vi "Act On Test.vi"(6 "Report Action":T1, 8 "error in":errorcluster, 9 "Values":variant[](array[variant]), 10 "Parameters":string[](array[string]), 11 "TDMS in":refnum<class "TDMS.lvclass">) -> (0 "error out":errorcluster, 3 "TDMS out":refnum<class "TDMS.lvclass">)   [LabVIEW 2019, in "TDMS.lvlib" / "TDMS.lvclass"]
uses:
  TDMS.lvclass
  builds/Tools/Report.lvlibp/Custom Controls/Report Action.ctl
  TDMS.lvclass/TDMS.ctl
  builds/Tools/Report.lvlibp/Report.lvclass
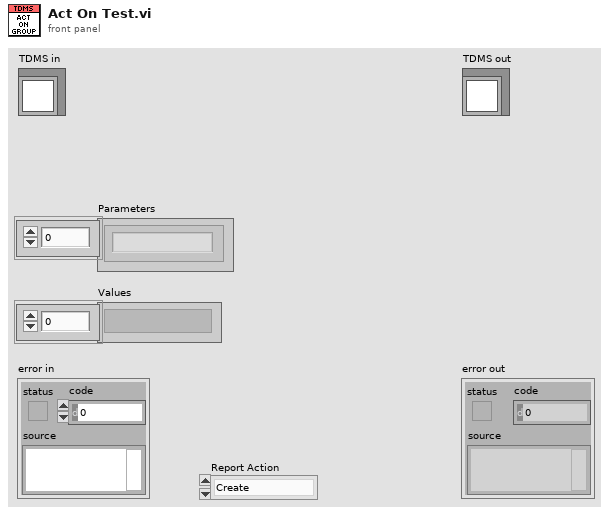
[diagram p1: front panel]
types:
  T1 = typedef "Report.lvlibp/Report.lvclass/Report Action.ctl" = enum16{"Create", "Append", "Destroy"}
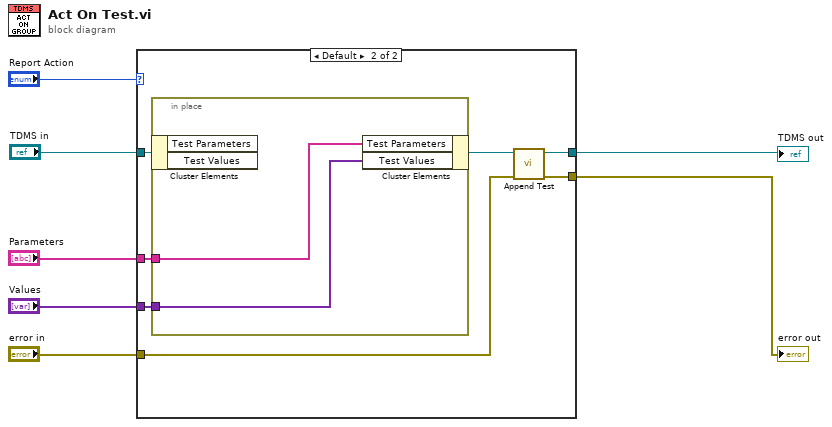
[diagram p0: block diagram]
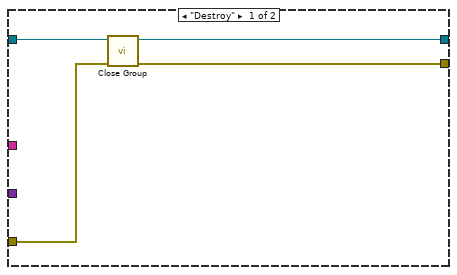
[diagram p2: hidden frame]
diagram:
  n1 = case shown="Default" "Report Action" {
    tunnel: "TDMS in" -> [w11 w18]
    tunnel: "Parameters" -> [_ w17]
    tunnel: "Values" -> [_ w16]
    tunnel: "error in" -> [w10 w12]
    tunnel: [w9 w14] -> w2
    tunnel: [w8 w13] -> w1
    frame "Destroy" {
      n2 = call "Close Group.vi"("error in"=w10, "TDMS in"=w11) -> ("error out"=w8:errorcluster, "TDMS out"=w9:refnum<class "TDMS.lvclass">)  [unwired: 8 in]
    }
    frame Default {
      n3 = in-place {
        in-place-border: w17 -> [w20]
        in-place-border: w16 -> [w19]
        n4 = in-place-cluster #1(w18) -> ()  [unwired: 2 out]
        n5 = in-place-cluster #1("Test Parameters"=w20, "Test Values"=w19) -> (w15:refnum<class "TDMS.lvclass">)
      }
      n6 = call "Append Test.vi"("error in"=w12, "TDMS in"=w15) -> ("error out"=w13:errorcluster, "TDMS out"=w14:refnum<class "TDMS.lvclass">)  [unwired: 8 in]
    }
  }
  "error out" <- w1
  "TDMS out" <- w2
